vi "pp3_DAQ_AudioClick.vi"(0 "State In":T1={"Curr  tr"=0, "Curr (ms)"=0, "Cum (ms)"=0, "Run loop diff"=0, "Tone countdown (ms)"=0, "Countdown (ms)"=0, "Curr State"=enum."0 NULL", "Prev State"=enum."1 Habituation", "Rw"=FALSE, "Sw"=FALSE, "Tone\nGate"=FALSE, "Punish"=FALSE, "Current DAQ DO Int"=0, "Current Loaded Trial"={"Trial Type Number"=1, "Trial Type"=enum."GO", "Trial Weight"=100, "Shock (mA)"=0.3, "Duration (ms)"=0.25, "Sound Type"=enum."04 FM Sweep", "Stim P1"=4000.0, "Stim P2"=0.0, "Stim P3"=0.0, "Stim P4"=2000.0, "DAQ Amplitude (V)"=0.25}, "Next Trial (for display purposes)"={"Trial Type Number"=1, "Trial Type"=enum."GO", "Trial Weight"=100, "Shock (mA)"=0.3, "Duration (ms)"=0.25, "Sound Type"=enum."04 FM Sweep", "Stim P1"=4000.0, "Stim P2"=0.0, "Stim P3"=0.0, "Stim P4"=2000.0, "DAQ Amplitude (V)"=0.25}, "Total trials memo"=0, "State start cum memo (ms)"=0, "Last dur jump time memo (ms)"=0, "Last dur shock time memo (ms)"=0, "Tone repeat memo (ms)"=0, "Webcam on"=FALSE, "Webcam recording"=FALSE, "State update flag"=FALSE, "Last loaded shock voltage"=0.0, "Vid upd"=enum."0"} {"Current DAQ DO Int" format="%016b"; "Next Trial (for display purposes)"."DAQ Amplitude (V)" min=0.0 max=5.0 format="%_4g"; "Next Trial (for display purposes)"."Shock (mA)" min=-1.0 max=5.0; "Next Trial (for display purposes)"."Trial Weight" step=1; "Next Trial (for display purposes)"."Duration (ms)" min=0.0 max=1.0; "Next Trial (for display purposes)"."Trial Type Number" min=1 max=256 step=1; "Current Loaded Trial"."DAQ Amplitude (V)" min=0.0 max=5.0 format="%_4g"; "Current Loaded Trial"."Shock (mA)" min=-1.0 max=5.0; "Current Loaded Trial"."Trial Weight" step=1; "Current Loaded Trial"."Duration (ms)" min=0.0 max=1.0; "Current Loaded Trial"."Trial Type Number" min=1 max=256 step=1}, 1 "Daq config":T6={"Sound AO"="Dev6/ao0", "Shock intesity AO"="Dev6/ao1", "Code_LED DO"="Dev6/port1:2", "Switch DI"="Dev6/port1/line0", "Webcam"="cam9", "Sound AO task"="", "Sound card task"=0, "Shock intensity AO task"="", "Code_LED DO task"="", "Switch DI task"="", "AO <=> Sound card"=FALSE, "Sound card"=0, "sample rate"=100000.0, "Variable shock"=TRUE, "Webcam on"=FALSE, "Waveform memo"={"t0"=timestamp(0 s since 1904-01-01), "dt"=1.0, "Y"=[]}, "Tone trigger"="PFI1", "Master-9 DO"="", "Master-9 DO task"="Dev6/port0/line5:7"} {"sample rate" min=8000.0; "Sound card task" format="%.0x"}, 2 "Pre click \n(V)":dbl, 3 "error in (no error)":errorcluster) -> (10 "error out":errorcluster)   [LabVIEW 2013]
uses:
  CTL_pp3c_DaqStatus.ctl
  <vilib>/userdefined/High Color/IMAQdx.ctl
  <vilib>/sound2/lvsound2.llb/Sound Output Task ID.ctl
  pp3_CTL_StateInfo.ctl
  pp3_CTL_State.ctl
  pp3_CTL_Trial.ctl
  pp3_CTL_TrialType.ctl
  labolabo2/waveforms/WFTypes.ctl
  <vilib>/DAQmx/write.llb/DAQmx Write (Analog Wfm 1Chan NSamp).vi
  <vilib>/sound2/lvsound2.llb/Sound Output Write (DBL Single).vi
  <vilib>/DAQmx/create/channels.llb/DAQmx Create Channel (AO-Voltage-Basic).vi
  <vilib>/DAQmx/configure/timing.llb/DAQmx Timing (Use Waveform).vi
  <vilib>/DAQmx/miscellaneous.llb/DAQmx Fill In Error Info.vi
  <resource>/objmgr/daqmx.rc
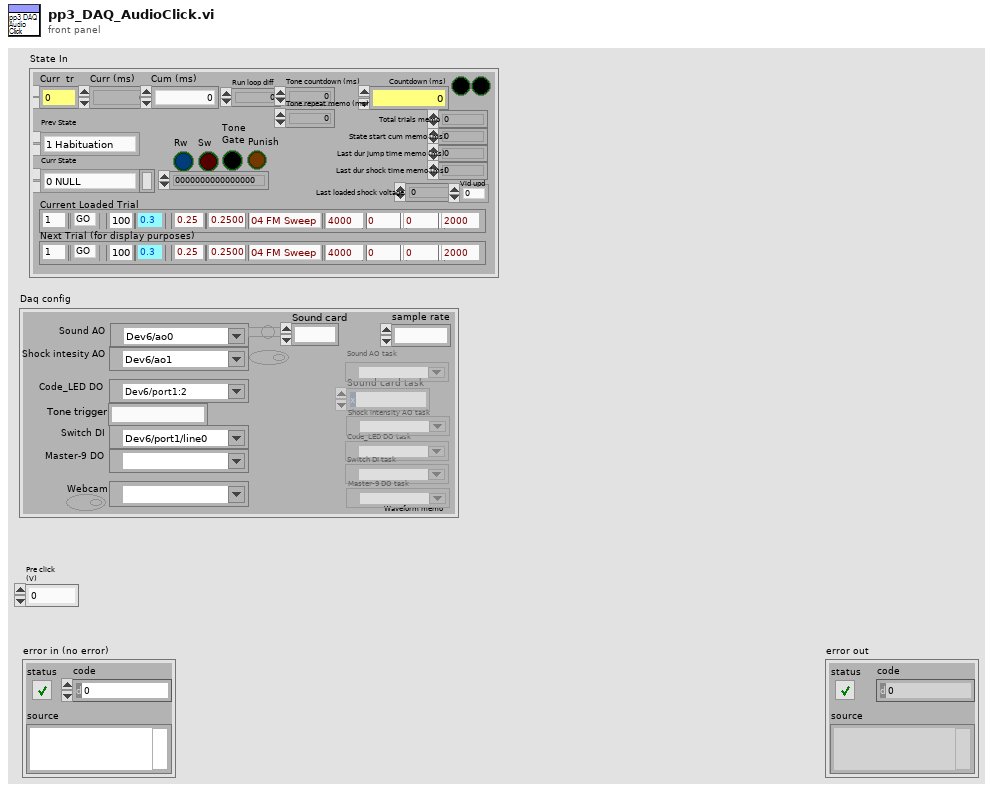
[diagram p1: front panel]
types:
  T1 = typedef "pp3_CTL_StateInfo.ctl" = cluster{"Curr  tr":u16, "Curr (ms)":u32, "Cum (ms)":i64, "Run loop diff":i64, "Tone countdown (ms)":i64, "Countdown (ms)":i64, "Curr State":T2, "Prev State":T2, "Rw":bool, "Sw":bool, "Tone\nGate":bool, "Punish":bool, "Current DAQ DO Int":u16, "Current Loaded Trial":T3, "Next Trial (for display purposes)":T3, "Total trials memo":i64, "State start cum memo (ms)":i64, "Last dur jump time memo (ms)":i64, "Last dur shock time memo (ms)":i64, "Tone repeat memo (ms)":i64, "Webcam on":bool, "Webcam recording":bool, "State update flag":bool, "Last loaded shock voltage":dbl, "Vid upd":enum16{"0", "1", "2", "3", "4", "5", "6", "7", "8", "9"}}
  T2 = typedef "pp3_CTL_State.ctl" = enum8{"0 NULL", "1 Habituation", "2 (Load Trial)", "3 Stay Period", "4 Load Audio/Click Delay", "5 GO Trial", "6 GO Jumped", "7 GO Timeout", "8 NOGO Trial", "9 NOGO Jumped", "10 NOGO Timeout", "11 TEST Trial", "12 TEST Jumped", "13 TEST Timeout", "14 Intertrial Interval", "15 Done"}
  T3 = typedef "pp3_CTL_Trial.ctl" = cluster{"Trial Type Number":i16, "Trial Type":T4, "Trial Weight":u32, "Shock (mA)":dbl, "Duration (ms)":dbl, "Sound Type":T5, "Stim P1":dbl, "Stim P2":dbl, "Stim P3":dbl, "Stim P4":dbl, "DAQ Amplitude (V)":dbl}
  T4 = typedef "pp3_CTL_TrialType.ctl" = enum16{"OFF", "GO", "NOGO", "TEST"}
  T5 = typedef "WFTypes.ctl" = enum16{"00 NULL", "01 DC", "02 Noise", "03 Pure Tone", "04 FM Sweep"}
  T6 = typedef "CTL_pp3c_DaqStatus.ctl" = cluster{"Sound AO":tag, "Shock intesity AO":tag, "Code_LED DO":tag, "Switch DI":tag, "Webcam":T7, "Sound AO task":refnum<k21>, "Sound card task":T8, "Shock intensity AO task":refnum<k21>, "Code_LED DO task":refnum<k21>, "Switch DI task":refnum<k21>, "AO <=> Sound card":bool, "Sound card":u32, "sample rate":dbl, "Variable shock":bool, "Webcam on":bool, "Waveform memo":waveform(dbl), "Tone trigger":string, "Master-9 DO":tag, "Master-9 DO task":refnum<k21>}
  T7 = typedef "IMAQdx.ctl" = refnum<k21>
  T8 = typedef "Sound Output Task ID.ctl" = u32
  T9 = typedef "pp2_CTL_DaqConfig.ctl" = cluster{"Sound AO":tag, "Shock intesity AO":tag, "Code_LED DO":tag, "Switch DI":tag, "Webcam":T7, "Sound AO task":refnum<k21>, "Sound card task":T8, "Shock intensity AO task":refnum<k21>, "Code_LED DO task":refnum<k21>, "Switch DI task":refnum<k21>, "AO <=> Sound card":bool, "Sound card":u32, "sample rate":dbl, "Variable shock":bool, "Webcam on":bool, "Tone gate PFI":tag, "Waveform memo":waveform(dbl), "First time":bool}
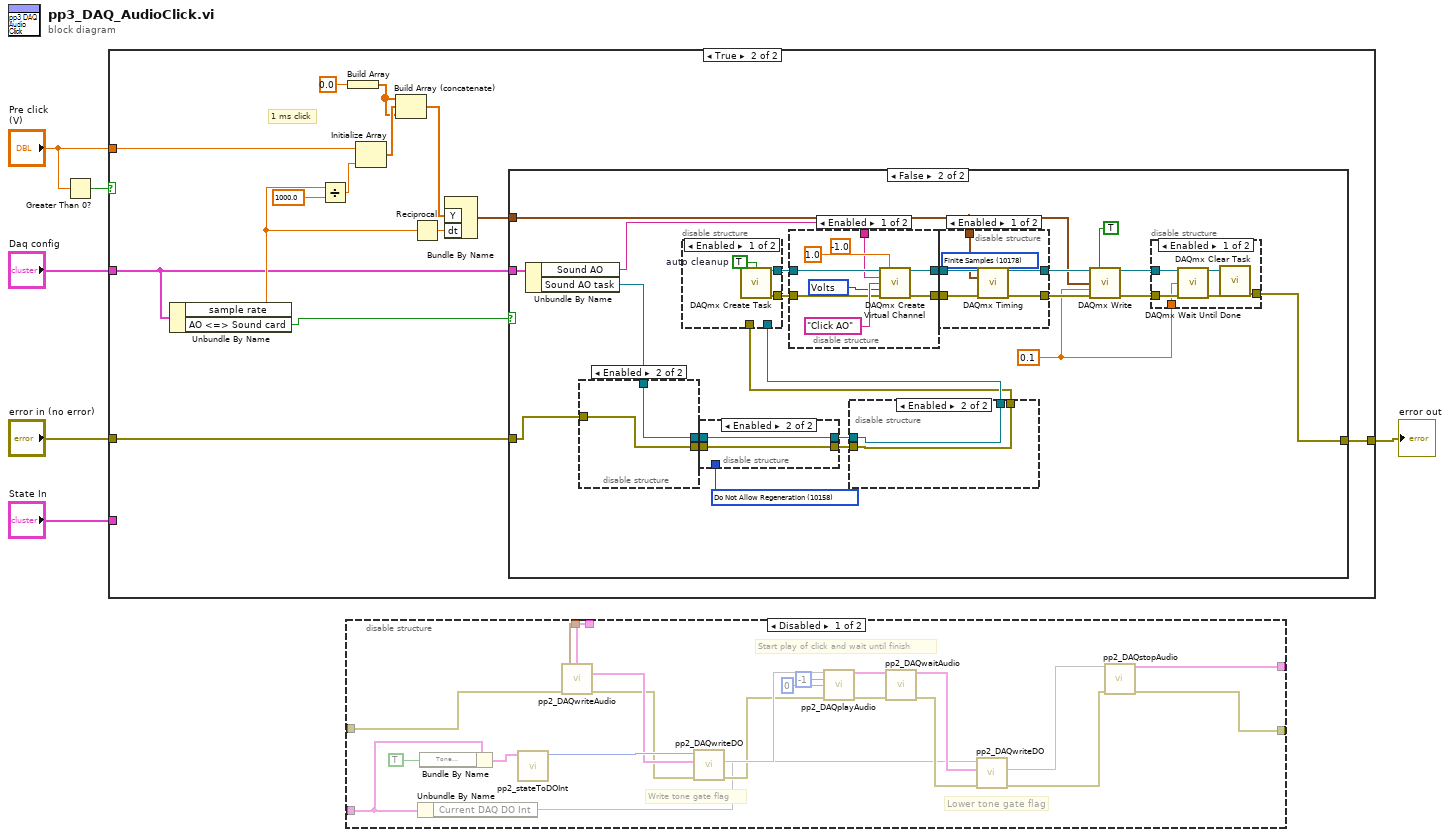
[diagram p0: block diagram]
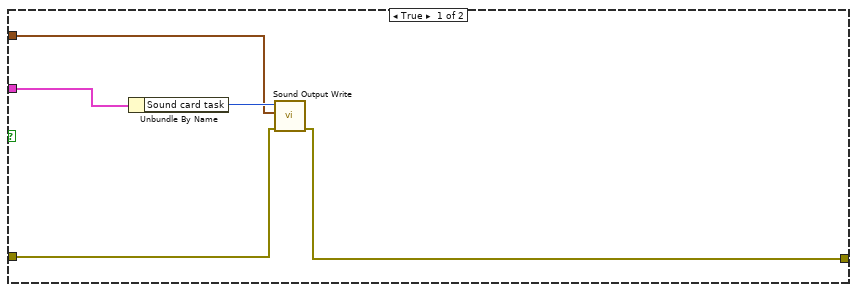
[diagram p4: hidden frame]
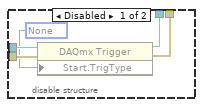
[diagram p5: hidden frame]
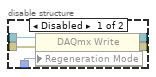
[diagram p6: hidden frame]
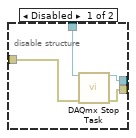
[diagram p7: hidden frame]
diagram:
  n1 = Greater Than 0?(x="Pre click \n(V)") -> (x > 0?=w3:bool)
  n2 = case shown="True" w3 {
    tunnel: "error in (no error)" -> [w7 w21]
    tunnel: [w7 w20] -> w5
    tunnel: "Daq config" -> [_ w9]
    tunnel: "Pre click \n(V)" -> [_ w11]
    tunnel: "State In" -> [_ _]
    frame False {
      # "If click amplitude is negative or zero, then just pass through without anything"
    }
    frame True {
      # "1 ms click"
      n3 = Unbundle By Name(w9) -> ("sample rate"=w14:dbl, "AO <=> Sound card"=w10:bool)
      n4 = Divide(x=w14, y=1000.0) -> (x/y=w16:dbl)
      n5 = Build Array(0.0 ("element")) -> (w17:dbl[])
      n6 = Initialize Array(w11, w16) -> (w19:dbl[])
      n7 = Build Array (concatenate)(w17, w19, w17) -> (w18:dbl[])
      n8 = Reciprocal(x=w14) -> (1/x=w13:dbl)
      n9 = Bundle By Name("Y"=w18, "dt"=w13) -> (w8:waveform(dbl))  [unwired: 1 in]
      n10 = case shown="False" w10 {
        tunnel: w21 -> [w26 w29]
        tunnel: [w25 w40] -> w20
        tunnel: w9 -> [w23 w37]
        tunnel: w8 -> [w22 w39]
        frame True {
          n11 = Unbundle By Name(w23) -> ("Sound card task"=w24:T8)
          n12 = call-poly <vilib>:"Sound Output Write.vi"("error in (no error)"=w26, "data"=w22, "task ID"=w24) -> ("error out"=w25:errorcluster)  [unwired: 7 in, 1 out]
        }
        frame False {
          w36 = 10158 items=["Allow Regeneration"=10097, "Do Not Allow Regeneration"=10158] ("RegenMode")
          w38 = 0.1 ("timeout")
          n13 = Unbundle By Name(w37) -> ("Sound AO"=w27:tag, "Sound AO task"=w28:refnum<k21>)
          n14 = disable-structure shown="Enabled" {
            disable-tunnel: [w67 w69] -> w31
            disable-tunnel: [w66 w68] -> w30
            disable-tunnel: w29 -> [w65 w68]
            disable-tunnel: w28 -> [w64 w69]
            frame Disabled {
              n15 = call <vilib>:"DAQmx Stop Task.vi"("task/channels in"=w64, "error in"=w65) -> ("task out"=w67:refnum<k21>, "error out"=w66:errorcluster)  [unwired: 12 in]
            }
            frame Enabled {
            }
          }
          n16 = disable-structure shown="Enabled" {
            disable-tunnel: w36 -> [w61 _]
            disable-tunnel: [w60 w63] -> w35
            disable-tunnel: [w59 w62] -> w34
            disable-tunnel: w31 -> [w58 w63]
            disable-tunnel: w30 -> [w57 w62]
            frame Disabled {
              n17 = property class="DAQmx Write"(reference=w58, error in=w57, "Regeneration Mode"=w61) -> (reference out=w60:refnum<k21>, error out=w59:errorcluster)
            }
            frame Enabled {
            }
          }
          n18 = disable-structure shown="Enabled" {
            disable-tunnel: w35 -> [w54 w56]
            disable-tunnel: w34 -> [w53 w55]
            disable-tunnel: [w51 w56] -> w33
            disable-tunnel: [w50 w55] -> w32
            frame Disabled {
              w52 = 10230 items=["Analog Level"=10101, "Analog Window"=10103, "Digital Level"=10152, "Digital Pattern"=10398, "None"=10230] ("Pause.TrigType")
              n19 = property class="DAQmx Trigger"(reference=w54, error in=w53, "Start.TrigType"=w52) -> (reference out=w51:refnum<k21>, error out=w50:errorcluster)
            }
            frame Enabled {
            }
          }
          n20 = disable-structure shown="Enabled" {
            disable-tunnel: [w89 w92] -> w42
            disable-tunnel: [w88 w91] -> w41
            disable-tunnel: w33 -> [_ w92]
            disable-tunnel: w32 -> [_ w91]
            frame Enabled {
              w90 = TRUE  # auto cleanup
              n21 = call <vilib>:"DAQmx Create Task.vi"("auto cleanup"=w90) -> ("task out"=w89:refnum<k21>, "error out"=w88:errorcluster)  [unwired: 13 in]
            }
            frame Disabled {
            }
          }
          n22 = disable-structure shown="Enabled" {
            disable-tunnel: [w82 w87] -> w49
            disable-tunnel: [w81 w86] -> w48
            disable-tunnel: w42 -> [w80 w87]
            disable-tunnel: w41 -> [w79 w86]
            disable-tunnel: w27 -> [w78 _]
            frame Enabled {
              w83 = 10348 items=["Volts"=10348, "From Custom Scale"=10065] ("units")
              (unwired) -1.0 ("minimum value")
              n23 = call-poly <vilib>:"DAQmx Create Virtual Channel.vi"("task in"=w80, "maximum value"=1.0, "physical channels"=w78, "name to assign"="Click AO", "units"=w83, "error in"=w79) -> ("task out"=w82:refnum<k21>, "error out"=w81:errorcluster)  [unwired: 8 in]
            }
            frame Disabled {
            }
          }
          n24 = disable-structure shown="Enabled" {
            disable-tunnel: w49 -> [w74 w77]
            disable-tunnel: w48 -> [w73 w76]
            disable-tunnel: [w72 w77] -> w47
            disable-tunnel: [w71 w76] -> w46
            disable-tunnel: w39 -> [w70 _]
            frame Enabled {
              w75 = 10178 items=["Finite Samples"=10178, "Continuous Samples"=10123, "Hardware Timed Single Point"=12522] ("sample mode")
              n25 = call-poly <vilib>:"DAQmx Timing.vi"("task/channels in"=w74, "sample mode"=w75, "waveform"=w70, "error in"=w73) -> ("task out"=w72:refnum<k21>, "error out"=w71:errorcluster)  [unwired: 10 in]
            }
            frame Disabled {
            }
          }
          n26 = call-poly <vilib>:"DAQmx Write.vi"("task/channels in"=w47, "auto start"=TRUE, "data"=w39, "timeout"=w38, "error in"=w46) -> ("task out"=w44:refnum<k21>, "error out"=w43:errorcluster)  [unwired: 8 in, 1 out]
          n27 = disable-structure shown="Enabled" {
            disable-tunnel: w44 -> [w98 _]
            disable-tunnel: w43 -> [w97 w99]
            disable-tunnel: [w94 w99] -> w40
            disable-tunnel: w38 -> [w93 _]
            frame Enabled {
              n28 = call <vilib>:"DAQmx Wait Until Done.vi"("task/channels in"=w98, "timeout (sec)"=w93, "error in"=w97) -> ("task out"=w96:refnum<k21>, "error out"=w95:errorcluster)  [unwired: 11 in]
              n29 = call <vilib>:"DAQmx Clear Task.vi"("task in"=w96, "error in"=w95) -> ("error out"=w94:errorcluster)  [unwired: 13 in]
            }
            frame Disabled {
            }
          }
        }
      }
    }
  }
  "error out" <- w5
  n30 = disable-structure shown="Disabled" {
    disable-tunnel: _ -> [w121 _]
    disable-tunnel: _ -> [w120 _]
    disable-tunnel: _ -> [w119 _]
    disable-tunnel: _ -> [w118 _]
    disable-tunnel: [w102 _] -> _
    disable-tunnel: [w100 _] -> _
    frame Disabled {
      # "Start play of click and wait until finish"
      # "Lower tone gate flag"
      # "Write tone gate flag"
      n31 = Unbundle By Name(w121) -> ("Current DAQ DO Int"=w106)
      n32 = Bundle By Name(cluster=w121, "Tone\nGate"=TRUE ("Tone\nGate")) -> (w117:cluster{})
      n33 = call "pp2_stateToDOInt.vi"("State In"=w117) -> ("DAQ Output Int"=w115:u16)  [unwired: 10 in]
      n34 = call "pp2_DAQwriteAudio.vi"("Daq config In"=w118, "Waveform"=w120, "error in (no error)"=w119) -> ("Daq config Out"=w105:T9, "error out"=w104:errorcluster)  [unwired: 11 in]
      n35 = call "pp2_DAQwriteDO.vi"("error in (no error)"=w104, "Daq config"=w105, "DAQ Digital In"=w115) -> ("error out"=w113:errorcluster, 2:w114)  [unwired: 7 in]
      n36 = call "pp2_DAQplayAudio.vi"("Daq config In"=w114, "State In"=i64 -1 ("Tone countdown (ms) In"), 7:i64 0 ("Tone repeat memo"), "error in (no error)"=w113) -> ("Daq config Out"=w110:T9, "error out"=w109:errorcluster)  [unwired: 9 in, 1 out]
      n37 = call "pp2_DAQwaitAudio.vi"("Daq config In"=w110, "error in (no error)"=w109) -> ("Daq config Out"=w107:T9, "error out"=w108:errorcluster)  [unwired: 12 in]
      n38 = call "pp2_DAQwriteDO.vi"("error in (no error)"=w108, "Daq config"=w107, "DAQ Digital In"=w106) -> ("error out"=w101:errorcluster, 2:w103)  [unwired: 7 in]
      n39 = call "pp2_DAQstopAudio.vi"("Daq config In"=w103, "error in (no error)"=w101) -> ("Daq config Out"=w102:T9, "error out"=w100:errorcluster)  [unwired: 12 in]
    }
    frame Enabled {
    }
  }
